vi "Link Channel.vi"(8 "error in (no error)":errorcluster, 11 "CIF_UI in":refnum<class "CIF_UI.lvclass">) -> (0 "error out":errorcluster, 3 "CIF_UI out":refnum<class "CIF_UI.lvclass">)   [LabVIEW 2021, in "CIF_UI.lvclass"]
uses:
  CIF_UI.lvclass
  CIF_UI.lvclass/CIF_UI.ctl
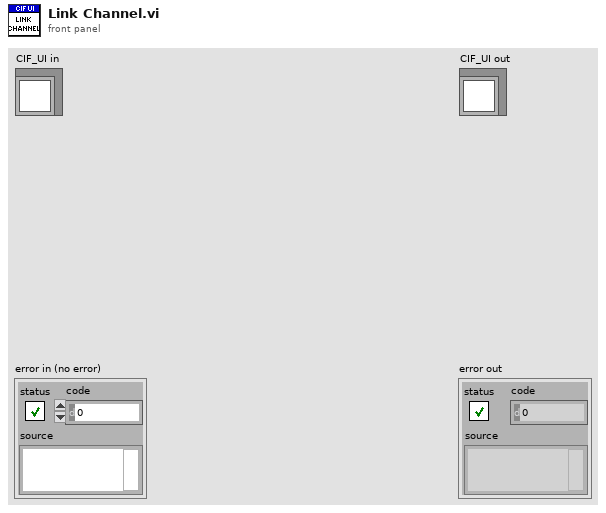
[diagram p1: front panel]
types:
  T1 = typedef "CIF_UI.lvclass/Channel Connection.ctl" = cluster{"Subscriber Name":string, "Publisher Name":string, "Custom Data":string}
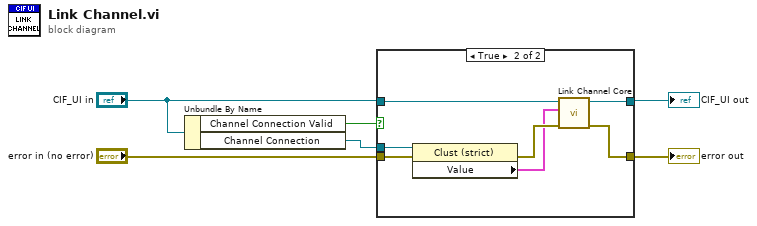
[diagram p0: block diagram]
diagram:
  n1 = Unbundle By Name("CIF_UI in") -> ("Channel Connection Valid"=w2:bool, "Channel Connection"=w1:refnum<vi>)
  n2 = case shown="True" w2 {
    tunnel: "error in (no error)" -> [w8 w15]
    tunnel: [w8 w10] -> w5
    tunnel: w1 -> [_ w14]
    tunnel: "CIF_UI in" -> [w7 w13]
    tunnel: [w7 w12] -> w3
    frame False {
    }
    frame True {
      n3 = property class="Clust (strict)"(reference=w14, error in=w15) -> (error out=w11:errorcluster, "Value"=w9:T1)  [unwired: 1 out]
      n4 = call "Link Channel Core.vi"("error in (no error)"=w11, "Channel Connection"=w9, "CIF_UI in"=w13) -> ("error out"=w10:errorcluster, "CIF_UI out"=w12:refnum<class "CIF_UI.lvclass">)  [unwired: 7 in]
    }
  }
  "error out" <- w5
  "CIF_UI out" <- w3
